vi "set_triggerable_flag.vi"(8 "error in (no error)":errorcluster, 10 "triggerable?":bool, 11 "SignalReaderDL091205FPGA in":refnum<class "SignalReaderDL091205FPGA.lvclass">) -> (0 "error out":errorcluster, 3 "SignalReaderDL091205FPGA out":refnum<class "SignalReaderDL091205FPGA.lvclass">)   [LabVIEW 2010, in "SignalReaderDL091205FPGA.lvclass"]
uses:
  SignalReaderDL091205FPGA.lvclass
  GenericSignalReader/GenericSignalReader/GenericSignalReader.lvclass
  SignalReaderDL091205FPGA.lvclass/SignalReaderDL091205FPGA.ctl
  FPGAWrapper/GenericFPGAWrapper/GenericFPGAWrapper/GenericFPGAWrapper.lvclass
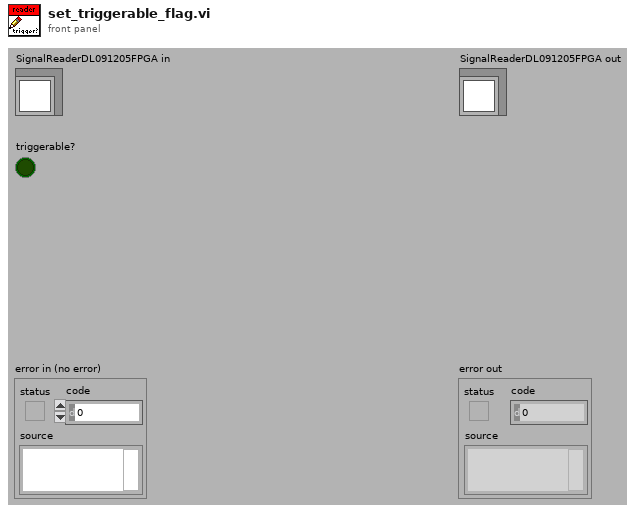
[diagram p1: front panel]
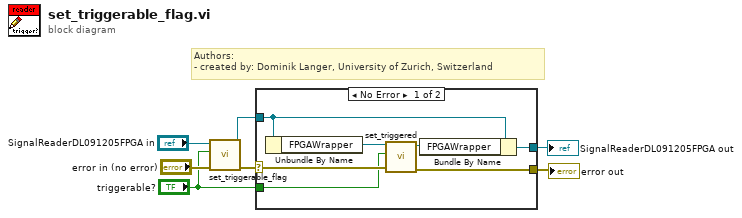
[diagram p0: block diagram]
diagram:
  # "Authors: \n- created by: Dominik Langer, University of Zurich, Switzerland"
  n1 = call-parent "set_triggerable_flag.vi"("error in (no error)"="error in (no error)", "triggerable?"="triggerable?", "GenericSignalReader in"="SignalReaderDL091205FPGA in") -> ("error out"=w5:errorcluster, "GenericSignalReader out"=w4:refnum<class "SignalReaderDL091205FPGA.lvclass">)  [unwired: 7 in]
  n2 = case shown="No Error" w5 {
    selector: w5 -> [w13 w15]
    tunnel: w4 -> [w14 w16]
    tunnel: "triggerable?" -> [w11 _]
    tunnel: [w10 w15] -> w2
    tunnel: [w8 w16] -> w1
    frame No Error {
      n3 = Unbundle By Name(w14) -> ("FPGAWrapper"=w12:refnum<class "GenericFPGAWrapper.lvclass">)
      n4 = call-dynamic "set_triggered.vi"("error in (no error)"=w13, "triggered?"=w11, "GenericFPGAWrapper in"=w12) -> ("error out"=w10:errorcluster, "GenericFPGAWrapper out"=w9:refnum<class "GenericFPGAWrapper.lvclass">)  [unwired: 7 in]
      n5 = Bundle By Name(cluster=w14, "FPGAWrapper"=w9) -> (w8:refnum<class "SignalReaderDL091205FPGA.lvclass">)
    }
    frame Error {
    }
  }
  "error out" <- w2
  "SignalReaderDL091205FPGA out" <- w1
